vi "StopSignal To DVR.vi"(1 "Refnum in":T1) -> (0 "Data Value Reference out":refnum<data-value>)   [LabVIEW 2017, in "StopSignal.lvlib"]
uses:
  StopSignal.lvlib
  Typedef/Def-StopSignalData.ctl
  Typedef/StopSignal.ctl
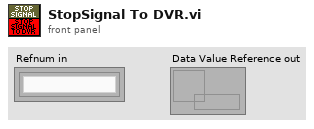
[diagram p1: front panel]
types:
  T1 = typedef "StopSignal.lvlib/StopSignal.ctl" = refnum<k1>
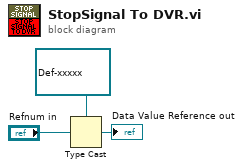
[diagram p0: block diagram]
diagram:
  n1 = Type Cast(type=refnum<data-value> refnum ("data value reference"), x="Refnum in") -> (*(type *) &x=→"Data Value Reference out":refnum<data-value>)
